vi "CommonVIs_GetFrontPanelControls.vi"(0 "OnlyControls(True)":bool=TRUE, 2 "error in (no error)":errorcluster) -> (14 "Event Registration Refnum":refnum<event-registration>, 15 "ControlRefs":refnum<vi>[](array[refnum]), 16 "error out":errorcluster)   [LabVIEW 2016]
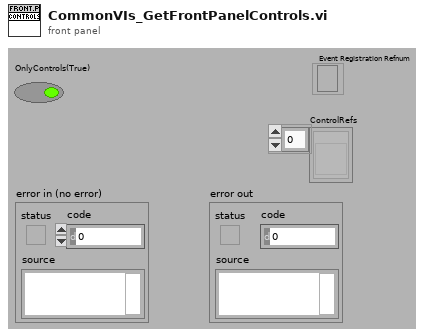
[diagram p1: front panel]
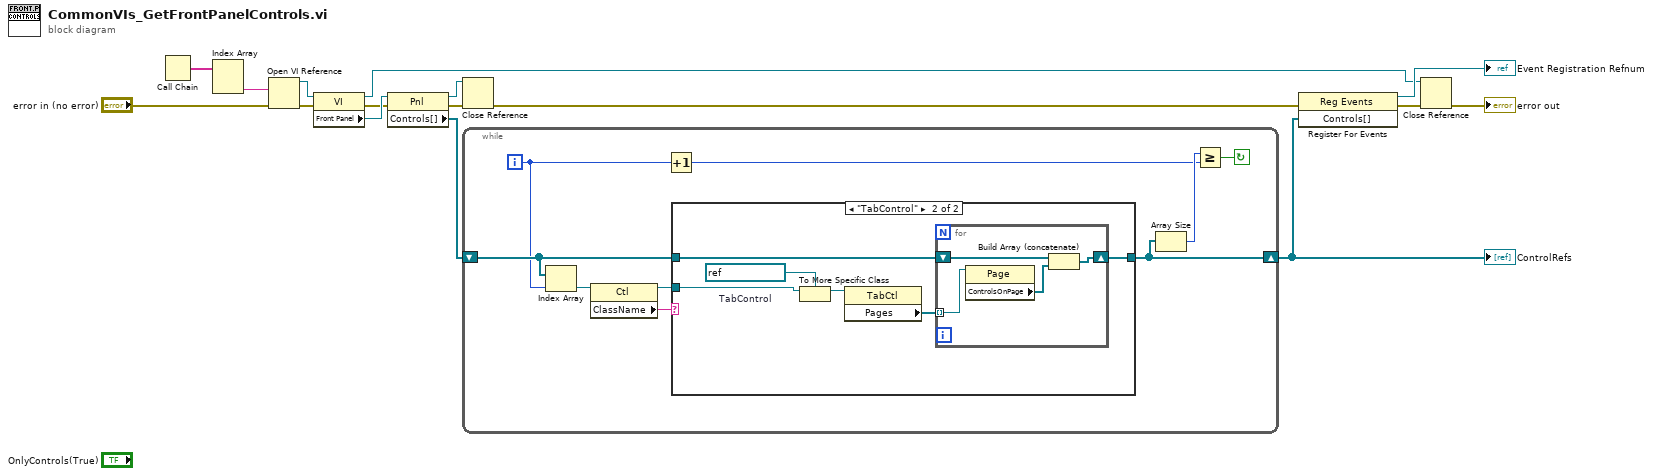
[diagram p0: block diagram]
diagram:
  n1 = Call Chain() -> (call chain=w9:string[])
  n2 = Index Array(array=w9) -> (element #2=w8:string)  [unwired: 2 in, 1 out]
  n3 = Open VI Reference(vi path=w8, error in (no error)="error in (no error)") -> (vi reference=w7:refnum<vi>, error out=w10:errorcluster)  [unwired: 4 out]
  n4 = property class="VI"(reference=w7, error in=w10) -> (reference out=w6:refnum<vi>, error out=w14:errorcluster, "Front Panel"=w15:refnum<vi>)
  n5 = property class="Pnl"(reference=w15, error in=w14) -> (reference out=w5:refnum<vi>, error out=w13:errorcluster, "Controls[]"=w2:refnum<vi>[])
  n6 = Close Reference(reference=w5, error in (no error)=w13) -> (error out=w12:errorcluster)
  n7 = while {
    shift-right: [w21] -> w1
    shift-left: w2 -> [w22]
    i -> [w19]
    stop <- w17 continue-if-true
    n8 = Index Array(array=w22, index=w19) -> (element=w23:refnum<vi>)
    n9 = property class="Ctl"(reference=w23) -> (reference out=w24:refnum<vi>, "ClassName"=w25:string)  [unwired: 1 in, 1 out]
    n10 = Increment(x=w19) -> (x+1=w18:i32)
    n11 = case shown="\"TabControl\"" w25 {
      tunnel: w24 -> [_ w32]
      tunnel: w22 -> [w26 w28]
      tunnel: [w26 w27] -> w21
      frame Default {
      }
      frame "TabControl" {
        w31 = refnum<vi> refnum  # TabControl
        n12 = To More Specific Class(target class=w31, reference=w32) -> (specific class reference=w30:refnum<vi>)  [unwired: 1 in, 1 out]
        n13 = property class="TabCtl"(reference=w30) -> ("Pages"=w29:refnum<vi>[])  [unwired: 1 in, 2 out]
        n14 = for {
          tunnel: w29 -> [w36] mode=indexing
          shift-right: [w33] -> w27
          shift-left: w28 -> [w35]
          n15 = property class="Page"(reference=w36) -> ("ControlsOnPage"=w34:refnum<vi>[])  [unwired: 1 in, 2 out]
          n16 = Build Array (concatenate)(w35, w34) -> (w33:refnum<vi>[])
        }
      }
    }
    n17 = Array Size(array=w21) -> (size(s)=w20:i32)
    n18 = Greater Or Equal?(x=w20, y=w18) -> (x >= y?=w17:bool)
  }
  "ControlRefs" <- w1
  n19 = register-events(error in=w12, w1) -> (reference out=→"Event Registration Refnum":refnum<event-registration>, error out=w4:errorcluster)  [unwired: 1 in]
  n20 = Close Reference(reference=w6, error in (no error)=w4) -> (error out=→"error out":errorcluster)
